vi "sqlbackup.vi"(8 "error in (no error)":errorcluster caption="错误输入（无错误）") -> (0 "error out":errorcluster caption="错误输出")   [LabVIEW 2016, in "数据查询.lvlib"]
uses:
  var/holding var.vi
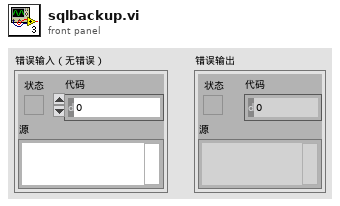
[diagram p1: front panel]
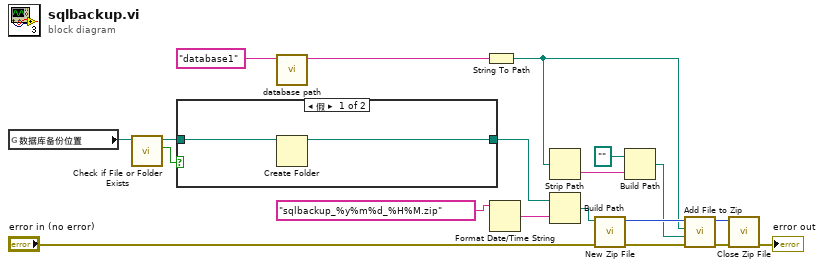
[diagram p0: block diagram]
diagram:
  n1 = global read "holding var.vi" "数据库备份位置"() -> (w6:path)
  n2 = call <vilib>:"Check if File or Folder Exists.vi"("path"=w6) -> ("file or folder exists?"=w5:bool, "dup path"=w4:path)  [unwired: 8 in, 1 out]
  n3 = case shown="假" w5 {
    tunnel: w4 -> [w21 w22]
    tunnel: [w20 w22] -> w3
    frame False {
      n4 = Create Folder(path (use dialog)=w21) -> (created path=w20:path)  [unwired: 2 in, 2 out]
    }
    frame True {
    }
  }
  n5 = call "database path.vi"("database"="database1") -> ("Path out"=w18:string)  [unwired: 9 in, 1 out]
  n6 = String To Path(string=w18) -> (path=w10:path)
  n7 = Format Date/Time String(time format string (%c)="sqlbackup_%y%m%d_%H%M.zip" ("时间格式字符串(%c)")) -> (date/time string=w12:string)  [unwired: 2 in]
  n8 = Strip Path(path=w10) -> (name=w9:string)  [unwired: 1 out]
  n9 = Build Path(base path=w3, name or relative path=w12) -> (appended path=w11:path)
  n10 = call <vilib>:"New Zip File.vi"("error in (no error)"="error in (no error)", "target"=w11) -> ("error out"=w15:errorcluster, "zip file out"=w17:i64)  [unwired: 3 in, 1 out]
  n11 = Build Path(base path=path "" ("基路径"), name or relative path=w9) -> (appended path=w7:path)
  n12 = call <vilib>:"Add File to Zip.vi"("error in (no error)"=w15, "destination path in zip"=w7, "source file path"=w10, "zip file in"=w17) -> ("error out"=w14:errorcluster, "zip file out"=w16:i64)  [unwired: 6 in]
  n13 = call <vilib>:"Close Zip File.vi"("error in (no error)"=w14, "zip file in"=w16) -> ("error out"=→"error out":errorcluster)  [unwired: 5 in]
